vi "CSM - Destroy Global Log Event.vi"(6 "timeout in ms (5000ms)":i32=5000, 8 "Error in":errorcluster caption="Error in (no error)", 9 "force Destroy?":bool, 11 "CSM Global Log Event":refnum<user-event>) -> (0 "Error out":errorcluster)   [LabVIEW 2020, in "Communicable State Machine.lvlib"]
doc: "Release CSM Global Log Event Reference.\n\n<b>Inputs:</b>\n - <b>CSM Global Log Event</b>:\n - <b>Error in</b>: Error cluster\n\n<b>Outputs:</b>\n - <b>Error out</b>: Error cluster"
uses:
  Communicable State Machine.lvlib
  _CSM_GlobalLog_MSG.ctl
  _CSM_Response Source Message.ctl
  _CSM_GlobalLog_MSG_TYPE.ctl
  GEvt-RequestDef.ctl
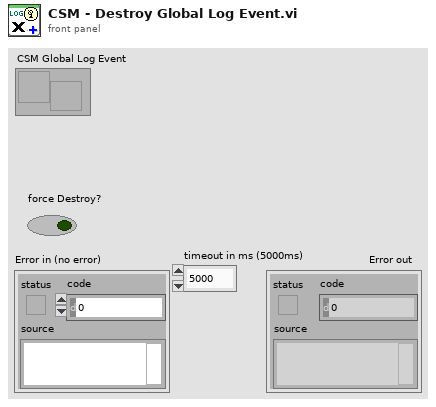
[diagram p1: front panel]
types:
  T1 = typedef "Communicable State Machine.lvlib/GEvt-RequestDef.ctl" = cluster{"Operation":enum16{"Obtain", "Destroy", "Force Destroy"}, "RespQ":refnum<queue>, "CSM Global Log Event":refnum<user-event>}
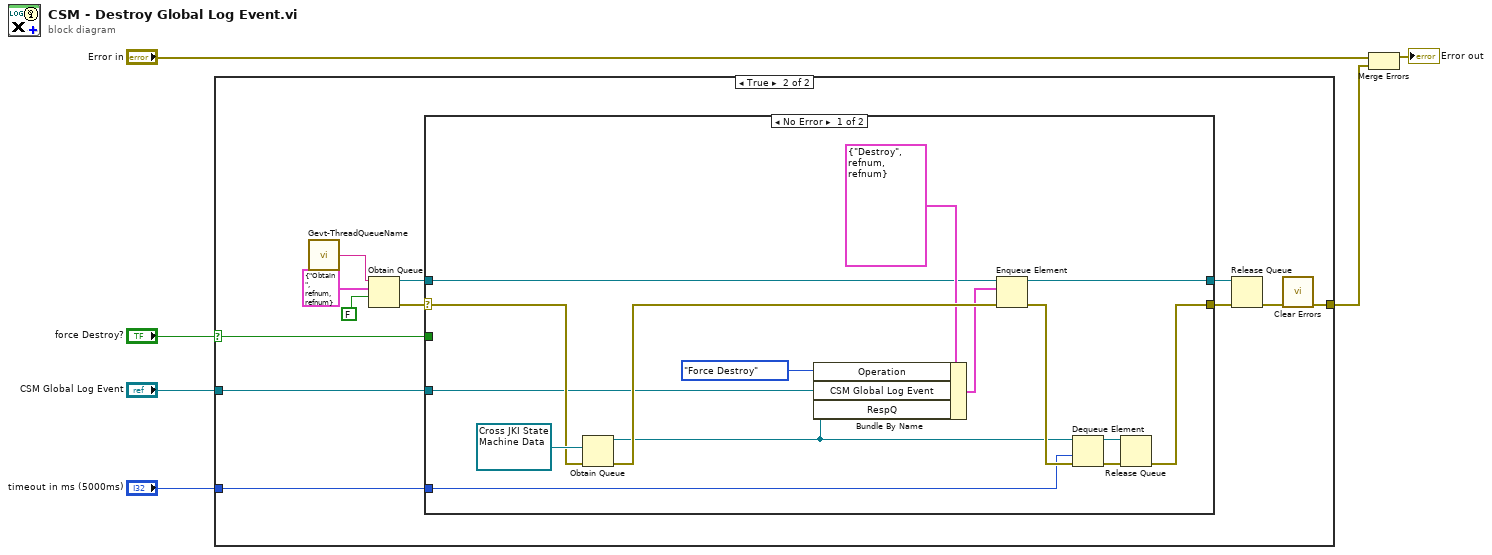
[diagram p0: block diagram]
diagram:
  n1 = case shown="True" "force Destroy?" {
    selector: "force Destroy?" -> [_ w16]
    tunnel: [_ w18] -> w4
    tunnel: "CSM Global Log Event" -> [_ w17]
    tunnel: "timeout in ms (5000ms)" -> [_ w15]
    frame False {
      # "For other case, watchdog thread will automatically free the event resource"
    }
    frame True {
      n2 = call "Gevt-ThreadQueueName.vi"() -> ("ThreadQueueName"=w7:string)  [unwired: 5 in]
      n3 = Obtain Queue(name (unnamed)=w7, element data type=T1 {"Operation"=enum."Obtain", "RespQ"=refnum, "CSM Global Log Event"=refnum}, create if not found? (T)=FALSE) -> (queue out=w11:refnum<queue>, error out=w12:errorcluster)  [unwired: 2 in, 1 out]
      n4 = case shown="No Error" w12 {
        selector: w12 -> [w24 w34]
        tunnel: w11 -> [w25 w35]
        tunnel: [w23 w35] -> w10
        tunnel: [w22 w34] -> w9
        tunnel: w17 -> [w21 _]
        tunnel: w16 -> [_ _]
        tunnel: w15 -> [w20 _]
        frame No Error {
          n5 = Obtain Queue(element data type=refnum<user-event> refnum ("CSM Global Log Event"), error in (no error)=w24) -> (queue out=w29:refnum<queue>, error out=w30:errorcluster)  [unwired: 3 in, 1 out]
          n6 = Bundle By Name(cluster=T1 {"Operation"=enum."Destroy", "RespQ"=refnum, "CSM Global Log Event"=refnum} ("element"), "Operation"=enum16{"Obtain", "Destroy", "Force Destroy"}."Force Destroy", "CSM Global Log Event"=w21, "RespQ"=w29) -> (w27:T1)
          n7 = Enqueue Element(queue=w25, element=w27, error in (no error)=w30) -> (queue out=w23:refnum<queue>, error out=w31:errorcluster)  [unwired: 1 in, 1 out]
          n8 = Dequeue Element(queue=w29, timeout in ms (-1)=w20, error in (no error)=w31) -> (queue out=w33:refnum<queue>, error out=w32:errorcluster)  [unwired: 2 out]
          n9 = Release Queue(queue=w33, error in (no error)=w32) -> (error out=w22:errorcluster)  [unwired: 1 in, 2 out]
        }
        frame Error {
        }
      }
      n10 = Release Queue(queue=w10, error in (no error)=w9) -> (error out=w8:errorcluster)  [unwired: 1 in, 2 out]
      n11 = call "Clear Errors.vi"("error in (no error)"=w8) -> ("error out"=w18:errorcluster)  [unwired: 5 in, 1 out]
    }
  }
  n12 = Merge Errors("Error in", w4) -> (→"Error out":errorcluster)
